vi "Transfer Controller.vi"(8 "error in":errorcluster) -> ()   [LabVIEW 2019]
doc: "This VI executes continuously carrying out the current operation and responding to updates or new operations. It will often contain the timing or control code that is difficult to place directly in TeleOp. This VI generally opens all sensors and motors and isolates the rest of the robot code from knowing how the operations are carried out."
uses:
  <vilib>/Rock Robotics/WPI/Framework/Completion Status.ctl
  Transfer Setpoints.ctl
  Transfer Operations.ctl
  <vilib>/Rock Robotics/WPI/ThirdParty/Phoenix-LabVIEW/Motor Controller/Controls/CTRE_Phoenix_MotorControl_NeutralMode.ctl
  <vilib>/Rock Robotics/WPI/ThirdParty/Phoenix-LabVIEW/Motor Controller/Controls/CTRE_Phoenix_MotorControl_ControlMode.ctl
  <vilib>/Rock Robotics/Network Tables/NT Write Boolean.vi
panel:
  in  "Interactive Values":T1
  out "Current\nCmd":string
  in  "Buttons":cluster{"Execute Cmd":bool, "Abort Cmd":bool}
  out "Command Timing":cluster{"Start Time (ms)":u32, "Iterations":i32}
  out "Status":T3
  # "Tip: It may be helpful to observe inputs and sensor values.\nYou may also want to display tuning or debugging controls."
  # "Interactive Command: You may fill in the settings for a command\nand schedule it with the Execute button. You can observe and abort\nany command while fine tuning the code for the controller."
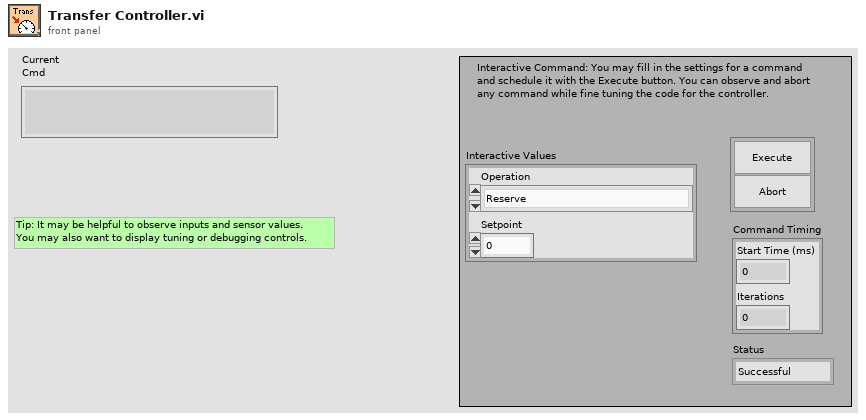
[diagram p1: front panel]
types:
  T1 = typedef "Transfer Setpoints.ctl" = cluster{"Operation":T2, "Setpoint":dbl}
  T2 = typedef "Transfer Operations.ctl" = enum16{"Reserve", "Read Current", "Immediate", "Shoot"}
  T3 = typedef "Completion Status.ctl" = enum16{"Successful", "Aborted", "Incomplete"}
  T4 = typedef "CTRE_Phoenix_MotorControl_NeutralMode.ctl" = enum8{"EEPROMSetting", "Override to Coast", "Override to Brake"}
  T5 = typedef "WPI_MotorControlDeviceRef.ctl" = cluster{"DeviceStatus":errorcluster, "Type":T6, "PWM":cluster{"PWM Channel":T7, "DeadBand":T8}, "CAN":cluster{"Device Number":u8, "SetOutput VI Ref":variant, "GetOutput VI Ref":variant, "Enable VI Ref":variant, "Disable VI Ref":variant, "Data":variant}, "Invert":bool, "DIO PWM":cluster{"PWM \"Enable\" Channel":T7, "DIOChannel":T9, "PWM Rate":dbl}}
  T6 = typedef "WPI_MotorControlType.ctl" = enum16{"PWM", "CAN", "DIO PWM"}
  T7 = typedef "FPGA_DIOPWMChannel.ctl" = enum8{"PWM 0", "PWM 1", "PWM 2", "PWM 3", "PWM 4", "PWM 5", "PWM 6", "PWM 7", "PWM 8", "PWM 9", "PWM MXP 0", "PWM MXP 1", "PWM MXP 2", "PWM MXP 3", "PWM MXP 4", "PWM MXP 5", "PWM MXP 6", "PWM MXP 7", "PWM MXP 8", "PWM MXP 9", "Invalid"}
  T8 = typedef "WPI_PWMDeadband.ctl" = cluster{"Name":string, "maxPositivePwm":i32, "minPositivePwm":i32, "centerPwm":i32, "maxNegativePwm":i32, "minNegativePwm":i32, "angularRange":u16}
  T9 = typedef "FPGA_DIOChannel.ctl" = enum8{"DIO 0", "DIO 1", "DIO 2", "DIO 3", "DIO 4", "DIO 5", "DIO 6", "DIO 7", "DIO 8", "DIO 9", "DIO MXP 0", "DIO MXP 1", "DIO MXP 2", "DIO MXP 3", "DIO MXP 4", "DIO MXP 5", "DIO MXP 6", "DIO MXP 7", "DIO MXP 8", "DIO MXP 9", "DIO MXP 10", "DIO MXP 11", "DIO MXP 12", "DIO MXP 13", "DIO MXP 14", "DIO MXP 15", "SPI Port CS1", "SPI Port CS2", "SPI Port CS3", "SPI Port MISO", "SPI Port MOSI", "Invalid"}
  T10 = typedef "Command Status Info.ctl" = cluster{"Name":string, "Status":T3, "notifier out":T11}
  T11 = typedef "Completion Notifier.ctl" = refnum<notifier>
  T12 = cluster{"Current Command":T1, "Command Timing":cluster{"Start Time (ms)":u32, "Iterations":i32}, "Command Arguments":cluster{"Command Info":T10, "Description":string, "Default Command":T1, "queue out":refnum<queue>, "Subsystem Name":string}}
  T13 = typedef "CTRE_Phoenix_MotorControl_ControlMode.ctl" = u16
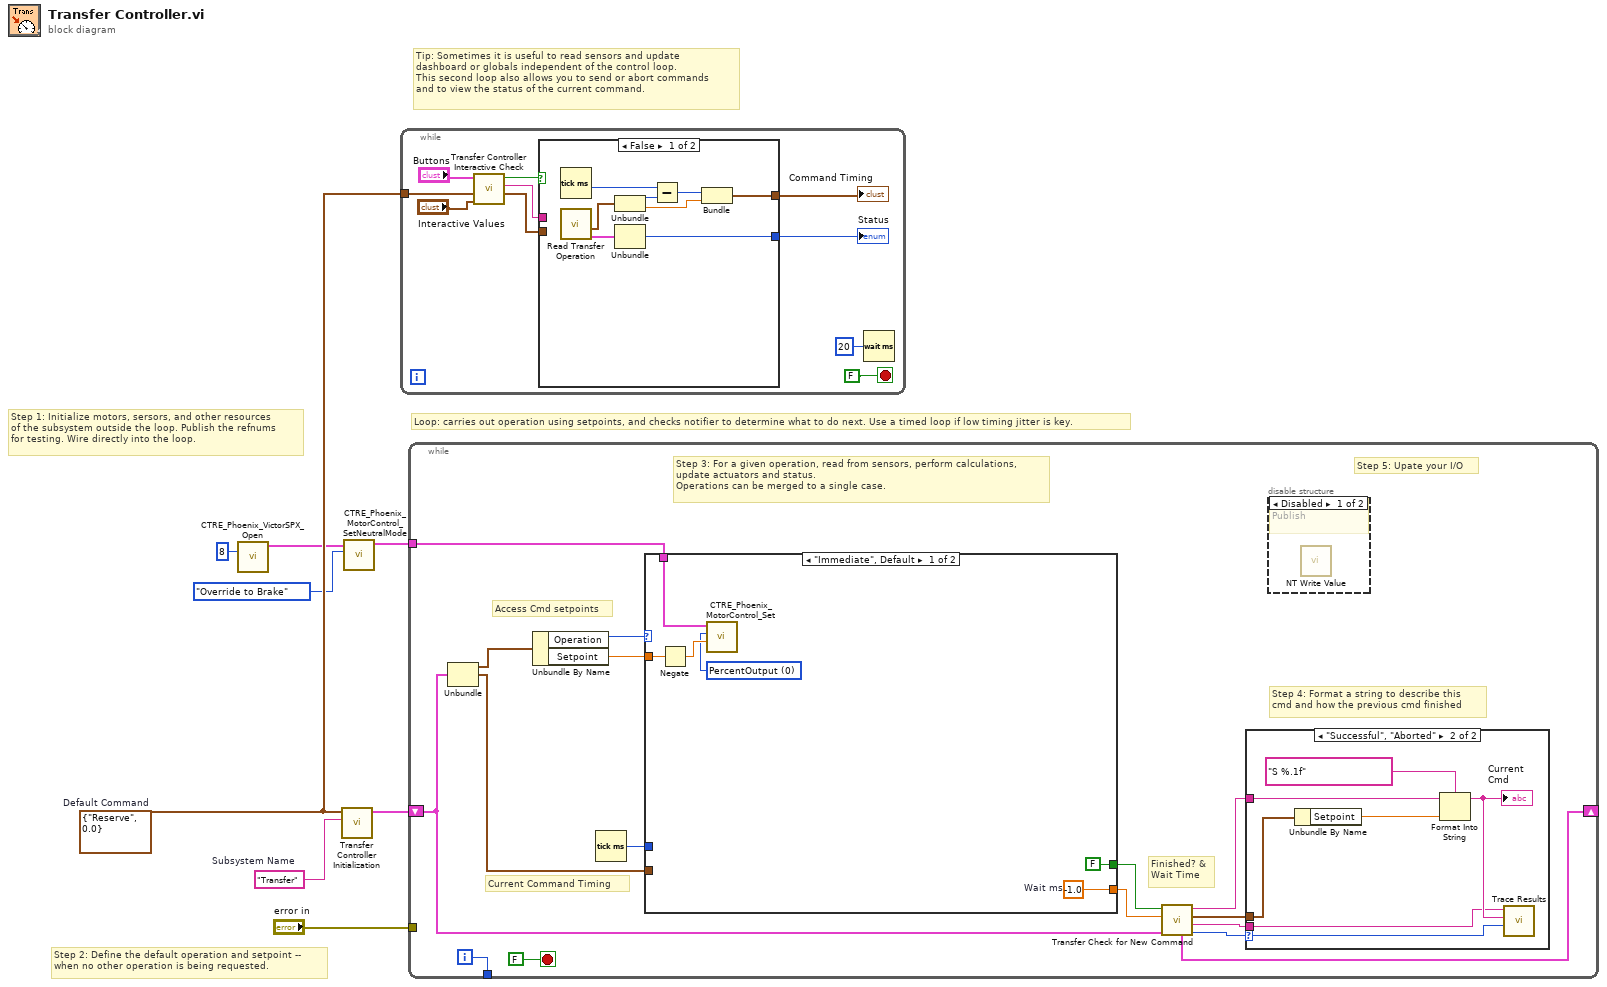
[diagram p0: block diagram]
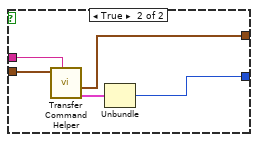
[diagram p2: hidden frame]
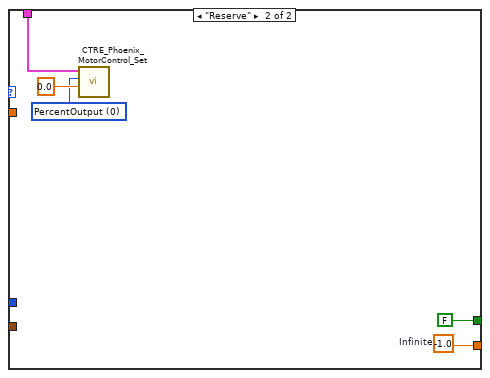
[diagram p5: hidden frame]
diagram:
  w5 = T1 {"Operation"=enum."Reserve", "Setpoint"=0.0}  # Default Command
  w6 = "Transfer"  # Subsystem Name
  # "Tip: Sometimes it is useful to read sensors and update\ndashboard or globals independent of the control loop.\nThis second loop also allows you to send or abort commands\nand to view the status of the current command."
  # "Step 2: Define the default operation and setpoint --\nwhen no other operation is being requested."
  # "Step 1: Initialize motors, sersors, and other resources\nof the subsystem outside the loop. Publish the refnums\nfor testing. Wire directly into the loop."
  # "Loop: carries out operation using setpoints, and checks notifier to determine what to do next. Use a timed loop if low timing jitter is key."
  n1 = call <vilib>:"CTRE_Phoenix_VictorSPX_Open.vi"("Device Number"=u8 8) -> ("CAN Talon SRX Ref"=w3:T5)  [unwired: 9 in, 1 out]
  n2 = call "Transfer Controller Initialization.vi"("Subsystem Name"=w6, "Default Command"=w5) -> ("Current Command"=w7:T12)  [unwired: 9 in]
  n3 = call <vilib>:"CTRE_Phoenix_MotorControl_SetNeutralMode.vi"("Motor Control Neutral Mode"=CTRE_Phoenix_MotorControl_NeutralMode."Override to Brake", "PhoenixMotorControlDevRef"=w3) -> ("PhoenixMotorControlDevRef"=w2:T5)  [unwired: 8 in, 1 out]
  n4 = while {
    tunnel: w5 -> [w15]
    stop <- FALSE stop-if-true
    n5 = call "Transfer Controller Interactive Check.vi"("Interactive Command in"="Interactive Values", "Default Command"=w15, "Buttons"="Buttons") -> ("Interactive Command out"=w12:T1, "Trace String"=w13:string, "Schedule"=w14:bool)  [unwired: 6 in]
    n6 = case shown="False" w14 {
      tunnel: [w26 w31] -> w11
      tunnel: w12 -> [_ w29]
      tunnel: [w22 w27] -> w10
      tunnel: w13 -> [_ w30]
      frame False {
        n7 = Tick Count (ms)() -> (millisecond timer value=w21:u32)
        n8 = call "Read Transfer Operation.vi"() -> ("Command Info"=w19:T10, "SubSystem Data"=w20:T1)  [unwired: 9 in, 1 out]
        n9 = Unbundle(w20) -> ("Operation"=w25:T2, "Setpoint"=w23:dbl)
        n10 = Unbundle(w19) -> ("Status"=w26:T3)  [unwired: 2 out]
        n11 = Subtract(x=w21, y=w25) -> (x-y=w24:u32)
        n12 = Bundle(w24, "Setpoint"=w23) -> (w22:cluster{u32, "Setpoint":dbl})  [unwired: 1 in]
      }
      frame True {
        n13 = call "Transfer Command Helper.vi"("Description"=w30, "SubSystem Data"=w29) -> ("Command Info Out"=w28:T10, "Command Timing"=w27:cluster{"Start Time (ms)":u32, "Iterations":i32})  [unwired: 7 in, 1 out]
        n14 = Unbundle(w28) -> ("Status"=w31:T3)  [unwired: 2 out]
      }
    }
    "Status" <- w11
    "Command Timing" <- w10
    n15 = Wait (ms)(milliseconds to wait=u32 20) -> ()  [unwired: 1 out]
  }
  n16 = while {
    shift-right: [w40] -> _
    shift-left: w7 -> [w33]
    tunnel: [w46] -> _
    tunnel: "error in" -> [_]
    tunnel: w2 -> [w32]
    i -> [w46]
    stop <- FALSE stop-if-true
    # "Step 5: Upate your I/O"
    # "Step 4: Format a string to describe this\ncmd and how the previous cmd finished"
    # "Current Command Timing"
    # "Access Cmd setpoints"
    # "Finished? &\nWait Time"
    # "Step 3: For a given operation, read from sensors, perform calculations,\nupdate actuators and status.\nOperations can be merged to a single case."
    n17 = Unbundle(w33) -> ("Current Command"=w45:T1, "Command Timing"=w42:cluster{"Start Time (ms)":u32, "Iterations":i32})  [unwired: 1 out]
    n18 = Unbundle By Name(w45) -> ("Operation"=w44:T2, "Setpoint"=w41:dbl)
    n19 = Tick Count (ms)() -> (millisecond timer value=w43:u32)
    n20 = case shown="\"Immediate\", Default" w44 {
      tunnel: [w60 w65] -> w38
      tunnel: [FALSE ("ignore previous (F)") FALSE ("ignore previous (F)")] -> w39
      tunnel: w42 -> [_ _]
      tunnel: w43 -> [_ _]
      tunnel: w41 -> [w58 _]
      tunnel: w32 -> [w59 w63]
      frame "Immediate", Default {
        w56 = T13 0 items=["PercentOutput"=0, "Position"=1, "Velocity"=2, "Current"=3, "Follower"=5, "MotionProfile"=6, "MotionMagic"=7, "MotionProfileArc"=10, "Disabled"=15] ("Control Mode")
        w60 = -1.0  # Wait ms
        n21 = Negate(x=w58) -> (-x=w57:dbl)
        n22 = call <vilib>:"CTRE_Phoenix_MotorControl_Set.vi"("Output"=w57, "Control Mode"=w56, "PhoenixMotorControlDevRef"=w59) -> ()  [unwired: 7 in, 2 out]
      }
      frame "Reserve" {
        w61 = T13 0 items=["PercentOutput"=0, "Position"=1, "Velocity"=2, "Current"=3, "Follower"=5, "MotionProfile"=6, "MotionMagic"=7, "MotionProfileArc"=10, "Disabled"=15] ("Control Mode")
        w65 = -1.0  # Infinite
        n23 = call <vilib>:"CTRE_Phoenix_MotorControl_Set.vi"("Output"=0.0, "Control Mode"=w61, "PhoenixMotorControlDevRef"=w63) -> ()  [unwired: 7 in, 2 out]
      }
    }
    n24 = call "Transfer Check for New Command.vi"("Current Command"=w33, "Wait time (ms)"=w38, "Finished?"=w39) -> ("Completion"=w34:T3, "Subsystem Name"=w35:string, "Current Command"=w36:T1, "Initial Trace String"=w37:string, "NextCommand"=w40:T12)  [unwired: 4 in]
    n25 = case shown="\"Successful\", \"Aborted\"" w34 {
      selector: w34 -> [_ w54]
      tunnel: w37 -> [_ w50]
      tunnel: w36 -> [_ w51]
      tunnel: w35 -> [_ w48]
      frame "Incomplete", Default {
        # "Continuing current command"
      }
      frame "Successful", "Aborted" {
        # "Report and setup for next command"
        n26 = Unbundle By Name(w51) -> ("Setpoint"=w53:dbl)
        n27 = Format Into String(format string="S %.1f", initial string=w50, w53) -> (resulting string=w49:string)  [unwired: 1 in, 1 out]
        "Current\nCmd" <- w49
        n28 = call <vilib>:"Trace Results.vi"("Status of previous command"=w54, "Description"=w49, "Subsystem"=w48) -> ()  [unwired: 9 in]
      }
    }
    n29 = disable-structure shown="Disabled" {
      frame Disabled {
        # "Publish"
        n30 = call-poly <vilib>:"NT Write Value.vi"() -> ()  [unwired: 11 in, 1 out]
      }
      frame Enabled {
      }
    }
  }
